vi "Remove Connection from State (data structure).vi"(8 "error in (no error)":errorcluster, 10 "Connection":T1, 11 "Routing State in":T2) -> (0 "error out":errorcluster, 1 "connection found":bool, 3 "Routing State out":T2)   [LabVIEW 2017, in "Switch Scripting.lvlib"]
uses:
  Switch Scripting.lvlib
  Routing State.ctl
  Connection.ctl
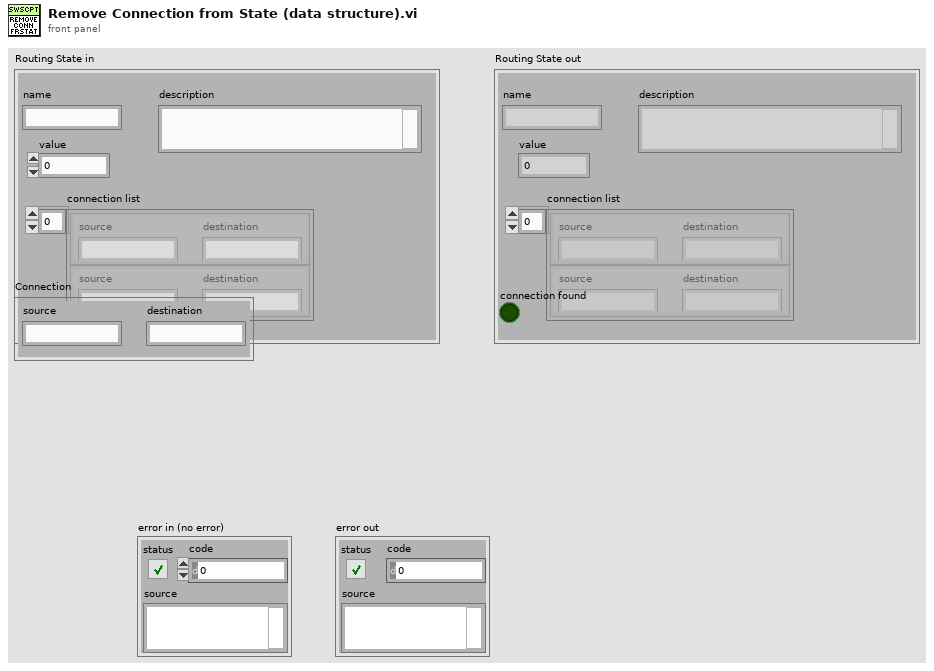
[diagram p1: front panel]
types:
  T1 = typedef "Switch Scripting.lvlib/Connection.ctl" = cluster{"source":string, "destination":string}
  T2 = typedef "Switch Scripting.lvlib/Routing State.ctl" = cluster{"name":string, "description":string, "value":i32, "connection list":T1[]}
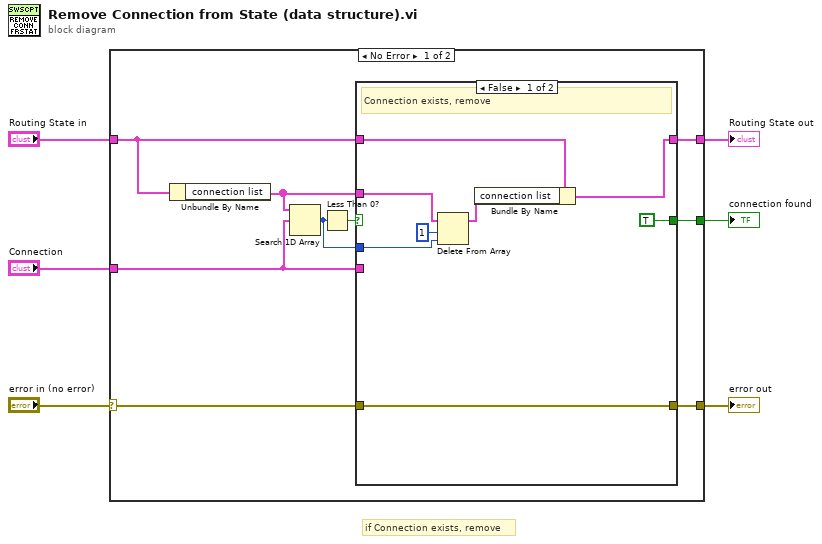
[diagram p0: block diagram]
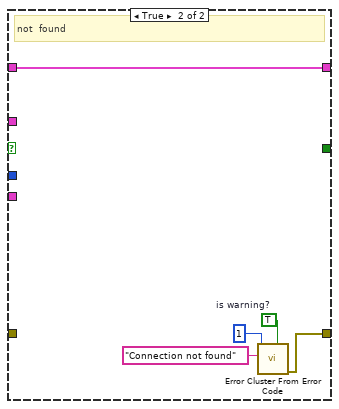
[diagram p2: hidden frame]
diagram:
  # "if Connection exists, remove"
  n1 = case shown="No Error" "error in (no error)" {
    selector: "error in (no error)" -> [w15 w30]
    tunnel: [w14 w30] -> w6
    tunnel: [w8 w29] -> w5
    tunnel: "Routing State in" -> [w9 w29]
    tunnel: "Connection" -> [w10 _]
    tunnel: [w12 _] -> w1
    frame No Error {
      n2 = Unbundle By Name(w9) -> ("connection list"=w11:T1[])
      n3 = Search 1D Array(1D array=w11, element=w10) -> (index of element=w7:i32)  [unwired: 1 in]
      n4 = Less Than 0?(x=w7) -> (x < 0?=w13:bool)
      n5 = case shown="False" w13 {
        tunnel: w15 -> [w16 _]
        tunnel: [w16 w24] -> w14
        tunnel: [TRUE _] -> w12
        tunnel: w11 -> [w22 _]
        tunnel: w10 -> [_ _]
        tunnel: w9 -> [w18 w28]
        tunnel: [w17 w28] -> w8
        tunnel: w7 -> [w20 _]
        frame False {
          # "Connection exists, remove"
          n6 = Delete From Array(array=w22, length=1, index=w20) -> (array with subset deleted=w19:T1[])  [unwired: 1 out]
          n7 = Bundle By Name(cluster=w18, "connection list"=w19) -> (w17:T2)
        }
        frame True {
          w26 = TRUE  # is warning?
          # "not  found"
          n8 = call <vilib>:"Error Cluster From Error Code.vi"("is warning? (False)"=w26, "error message (\"\")"="Connection not found" ("error message (\"\")"), "error code (0)"=1) -> ("error out"=w24:errorcluster)  [unwired: 6 in]
        }
      }
    }
    frame Error {
    }
  }
  "error out" <- w6
  "Routing State out" <- w5
  "connection found" <- w1
